vi "Gas-Control-GUI-v2.vi"() -> ()   [LabVIEW 2021]
uses:
  Controls/AR-Auto-Fill.ctl
  Controls/AR-Auto-Purge.ctl
  Controls/AR-DO-Action.ctl
panel:
  in  "Tab Control":enum32{"INDICATORS", "CHART"}(tab)
  out "Vac sol timer":dbl caption="Vac Solenoid Timer" format="%.1f sec"
  out "Gas sol timer":dbl caption="Gas Solenoid Timer" format="%.1f sec"
  out "O2 Timer":dbl format="%.1f sec"
  out "10 Torr (AI0)":dbl=10.152873763511888 caption="10 Torr Gage" format="%.3f Torr"
  out "1000 Torr (AI1)":dbl=821.8018332044094 caption="1000 Torr Gage" format="%.2f Torr"
  out "O2 1000ppm (AI3)":dbl=-245.94695681089067 caption="1000 PPM O2" format="%.0f PPM"
  out "0-25% O2 (AI2)":dbl=-6.135249063386897 caption="0-25% O2" format="%.2f %"
  in  "Full Ar Limit Torr":dbl=850.0 format="%#_13g"
  in  "Pump Down Limit Torr":dbl=320.0 format="%#_13g"
  in  "Partial Ar Fill Limit Torr":dbl=750.0 format="%#_13g"
  in  "Number of cycles":i32=25
  out "Cycle Timer":dbl format="%.1f sec"
  out "Completed Cycles":i32
  out "Pressure/O2":T1(graph) caption="Waveform Chart - Light"
  out "error out":errorcluster
  out "Log Written":bool=TRUE
  in  "Every X sec":dbl=60.0
  in  "Path to Save Report":path=path "C:/Users/cleanroom/Desktop/Gas-cycle-logs/Cycles-11-9-(750T-24cyc).csv"
  in  "LOG":bool
  out "Data":bool[](array[boolean])=[FALSE, FALSE, TRUE]
  in  "1000T Sim 2":dbl=1.0
  in  ">750 sim 2":bool=TRUE
  in  "10T Sim 2":dbl=10.0
  in  "<0.1T sim 2":bool
  out "Purge State":T2
  in  "simulate":bool
  out "Fill State":T3
  out "O2 pwr":bool
  out "Gas SOL":bool
  out "Vac SOL":bool
  in  "Quit":bool
  out "Purge Done":bool
  in  "Auto purge":bool
  out "Gage Err (DI2)":bool
  in  "O2 1000ppm (DO3)":bool
  in  "Gas sol (DO2)":bool
  in  "Vac sol (DO1)":bool
  in  "Pump (DO0)":bool
  out "Fill Done":bool
  in  "Auto fill":bool
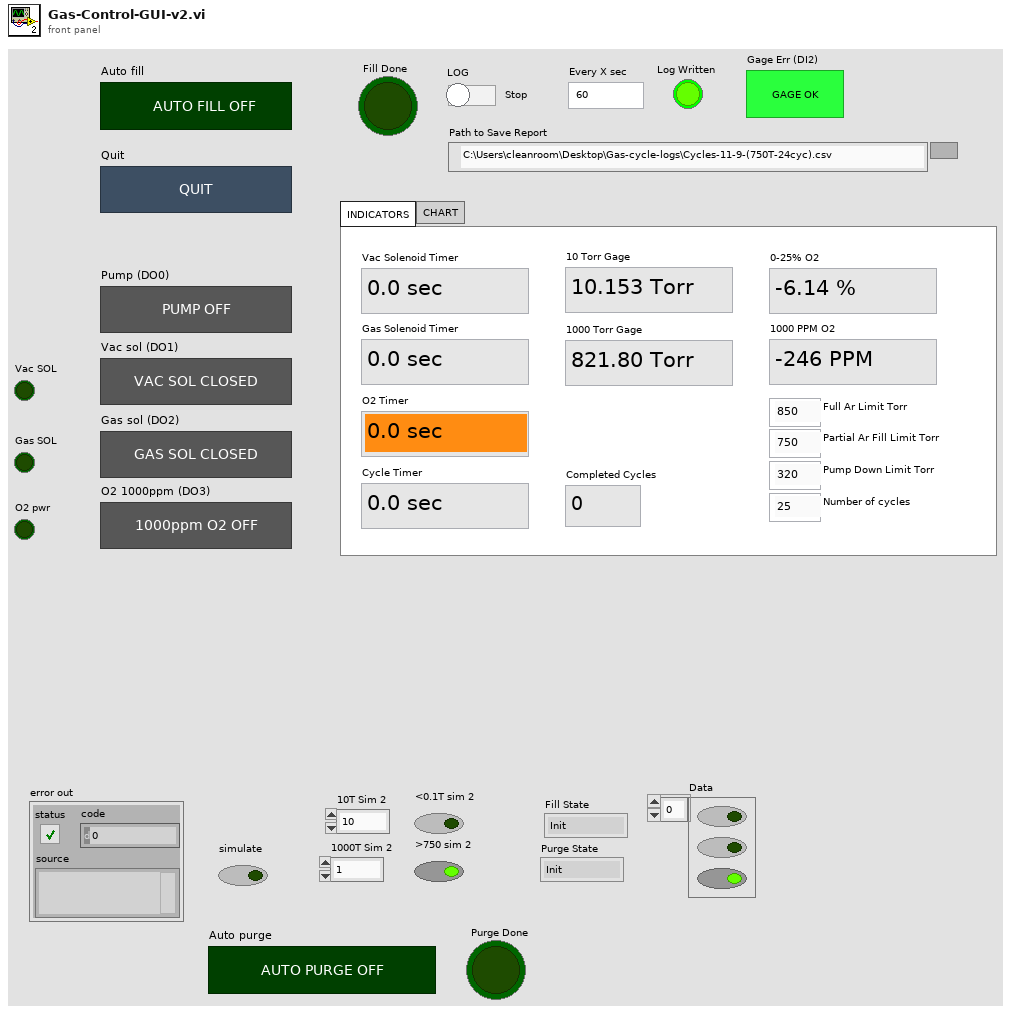
[diagram p1: front panel]
types:
  T1 = cluster{"1000 Torr (AI1)":dbl, "O2 1000ppm (AI3)":dbl}
  T2 = typedef "AR-Auto-Purge.ctl" = enum16{"Init", "Start Pump", "Stop Pump", "10T Gage", "1000T Gage", "End"}
  T3 = typedef "AR-Auto-Fill.ctl" = enum16{"Init", "Start Pump", "Stop Pump", "Gas Open", "Gas Close", "10T Gage", "1000T Gage", "End", "Vac Open", "Vac Close", "Decide"}
  T4 = typedef "AR-DO-Action.ctl" = enum16{"Init", "Update", "Keep DO3"}
  T5 = enum8{"Enabled", "Disabled", "Disabled and Grayed Out"}
  T6 = cluster{"10 Torr (AI0)":dbl, "1000 Torr (AI1)":dbl, "0-25% O2 (AI2)":dbl, "O2 1000ppm (AI3)":dbl, "Vac sol timer":dbl, "Gas sol timer":dbl, "O2 Timer":dbl, "Vac SOL":bool, "Gas SOL":bool, "O2 1000ppm (DO3)":bool}
  T7 = cluster{"1000 Torr (AI1)":dbl, "O2 1000ppm (AI3)":dbl}[]
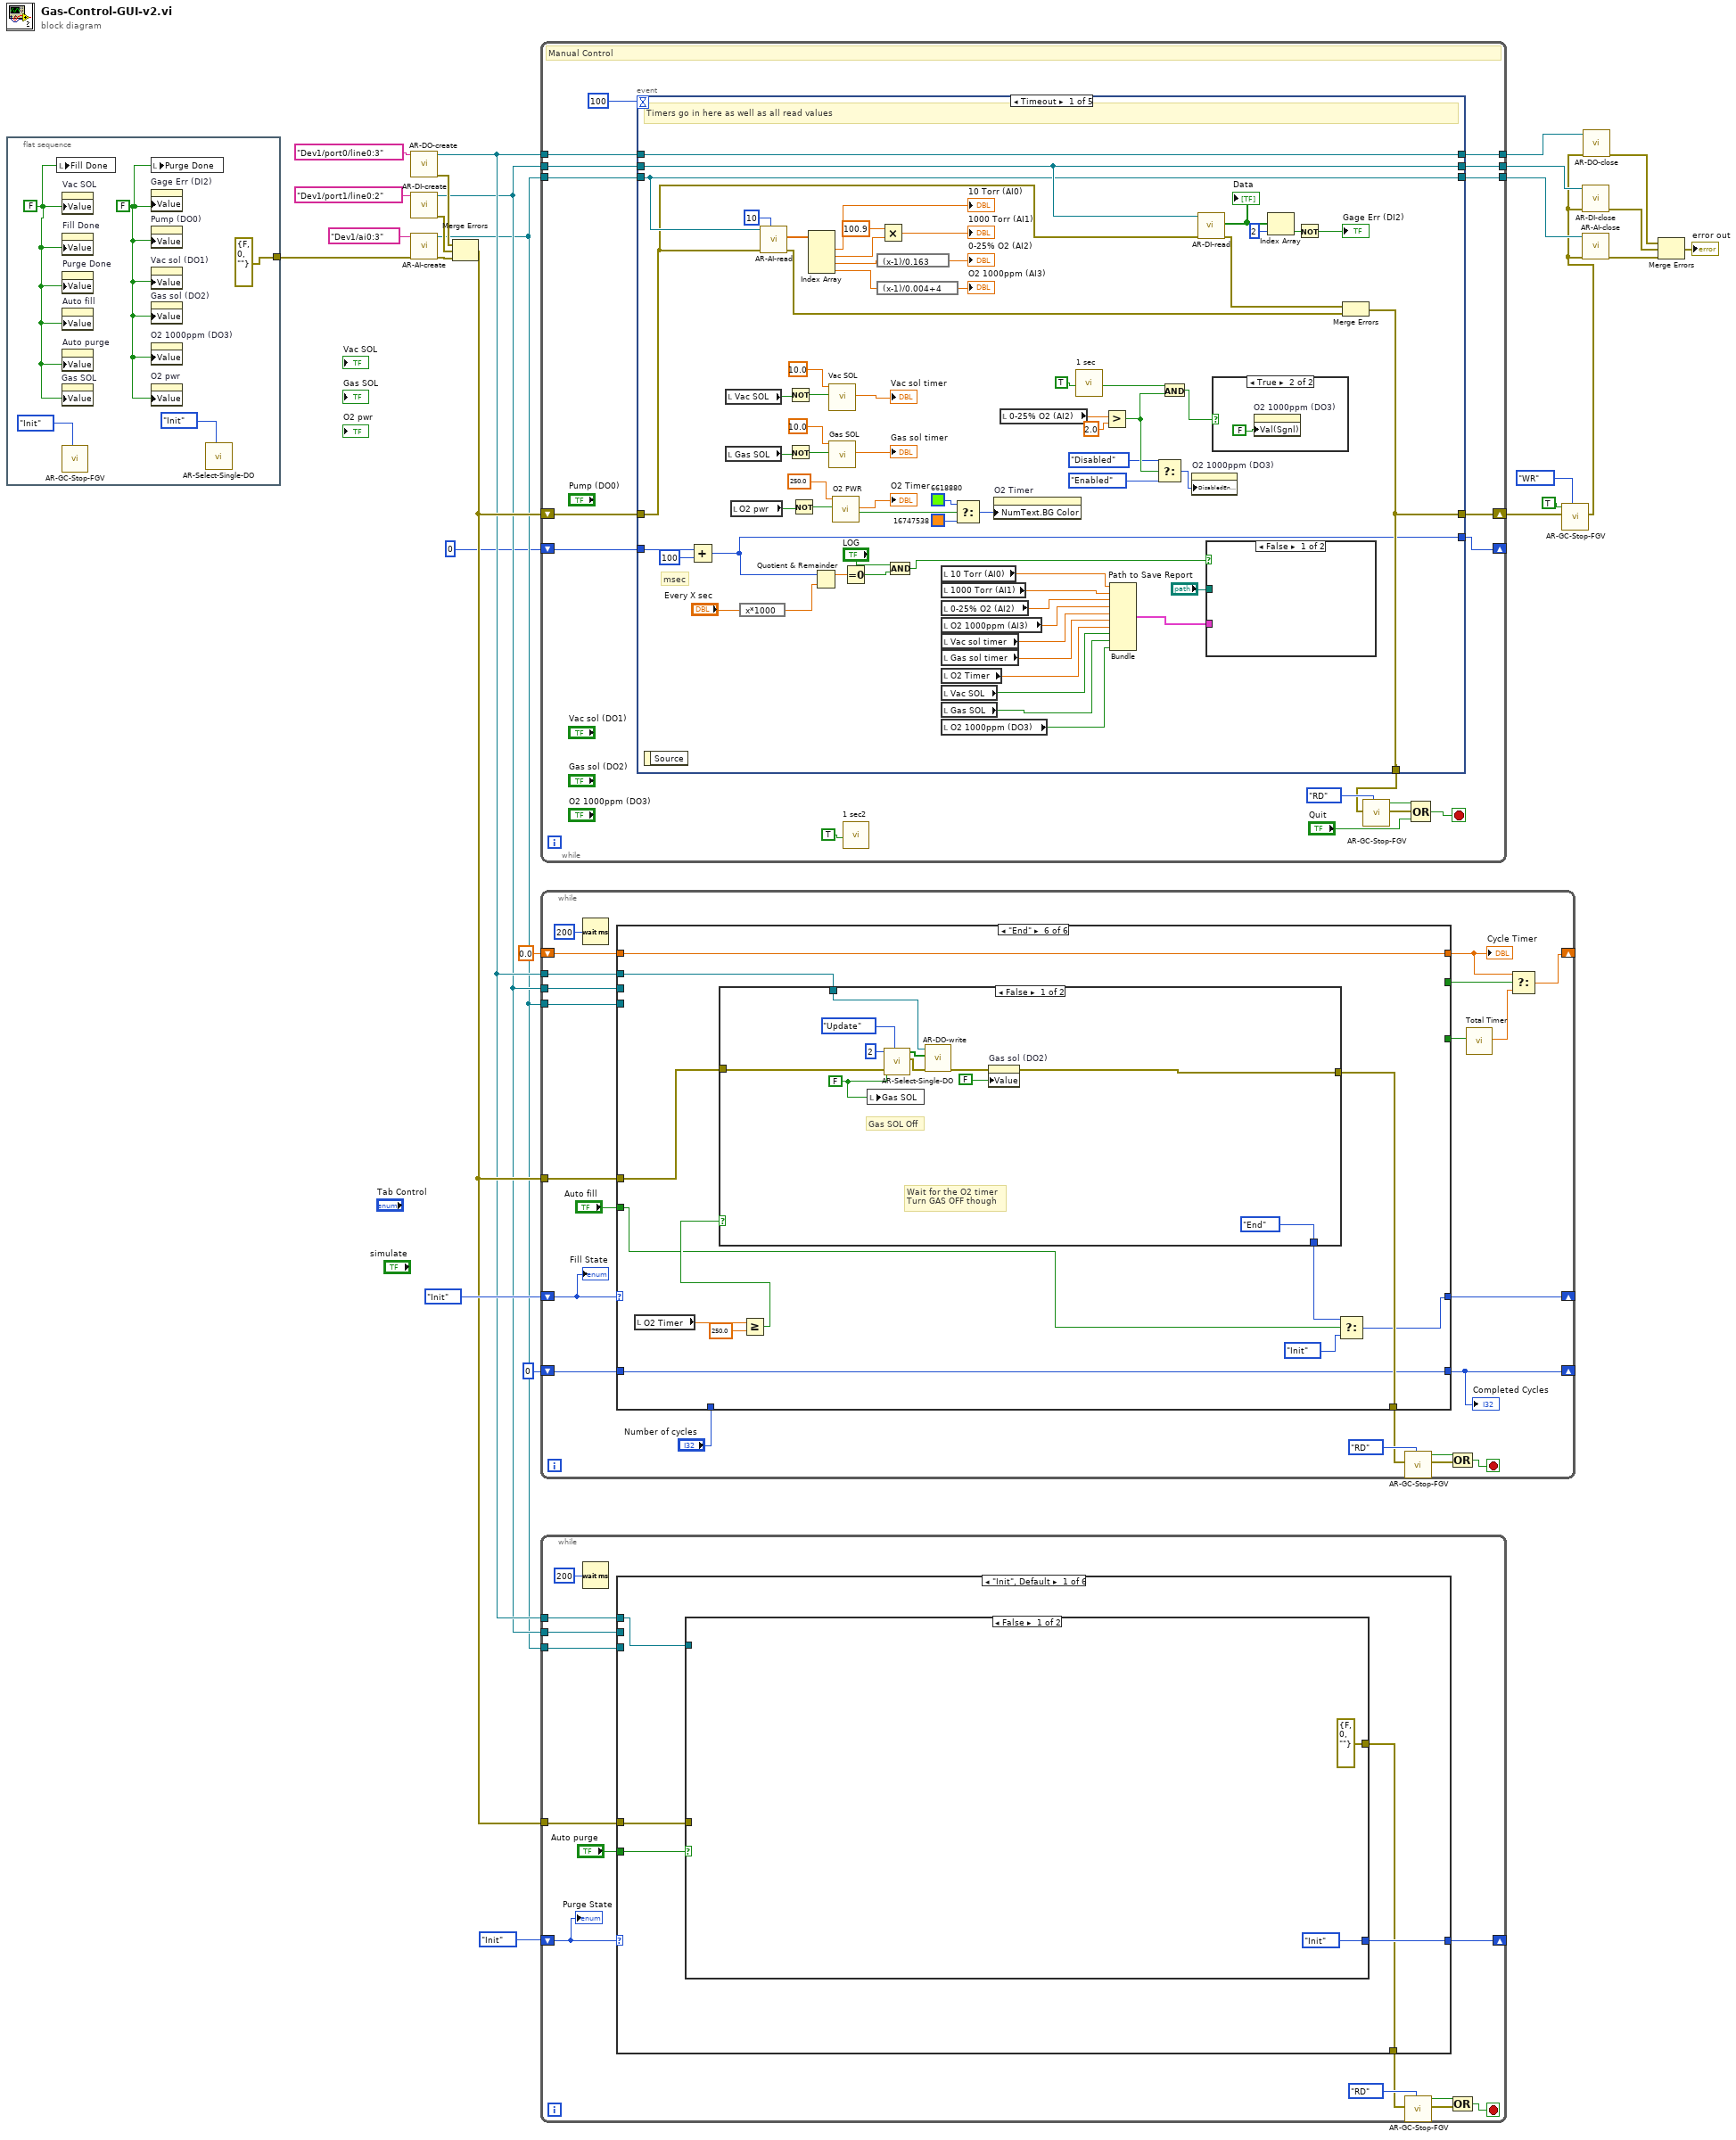
[diagram p0: block diagram]
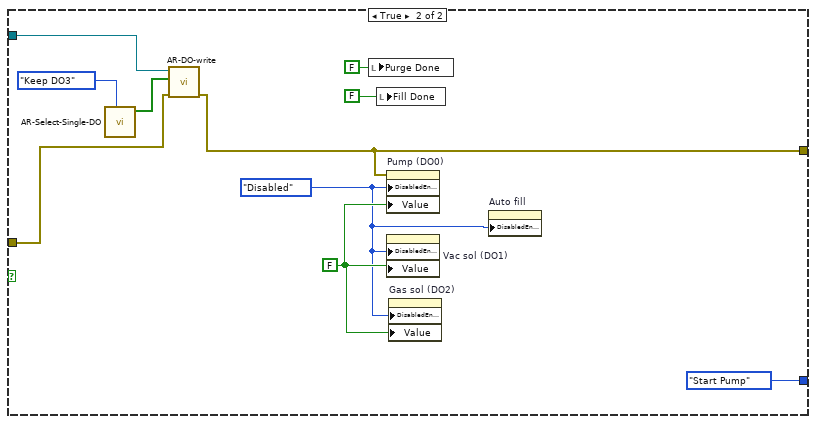
[diagram p2: hidden frame]
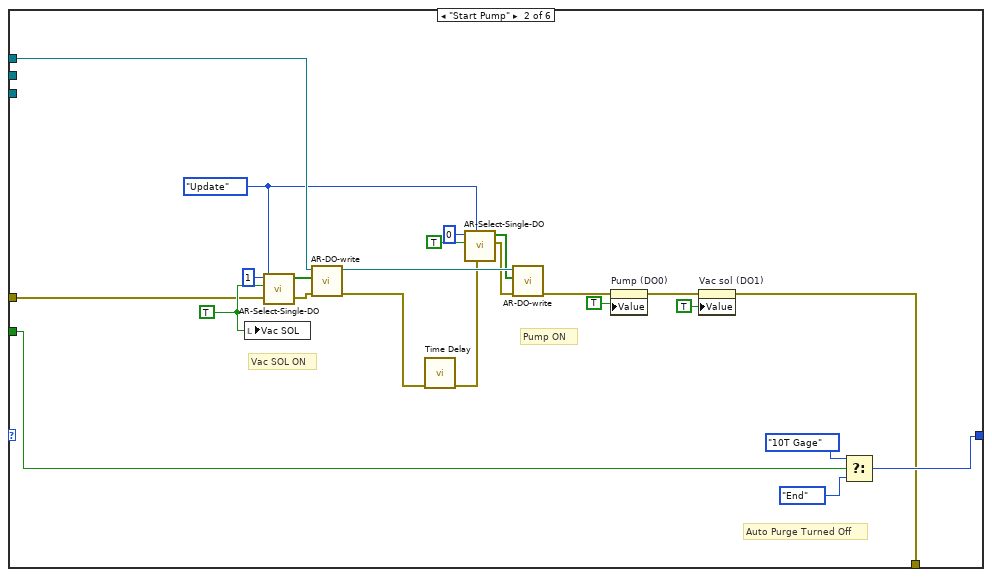
[diagram p3: hidden frame]
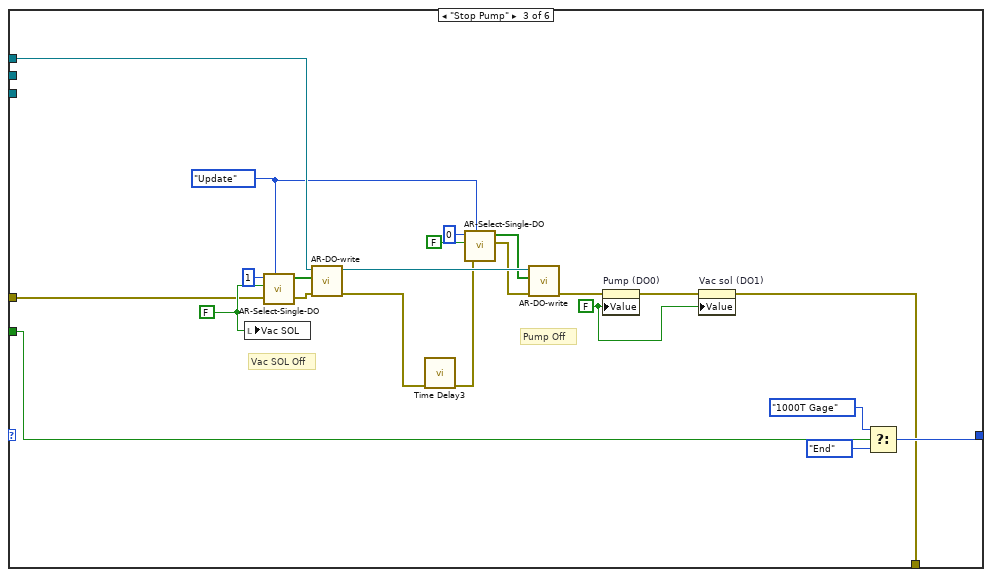
[diagram p4: hidden frame]
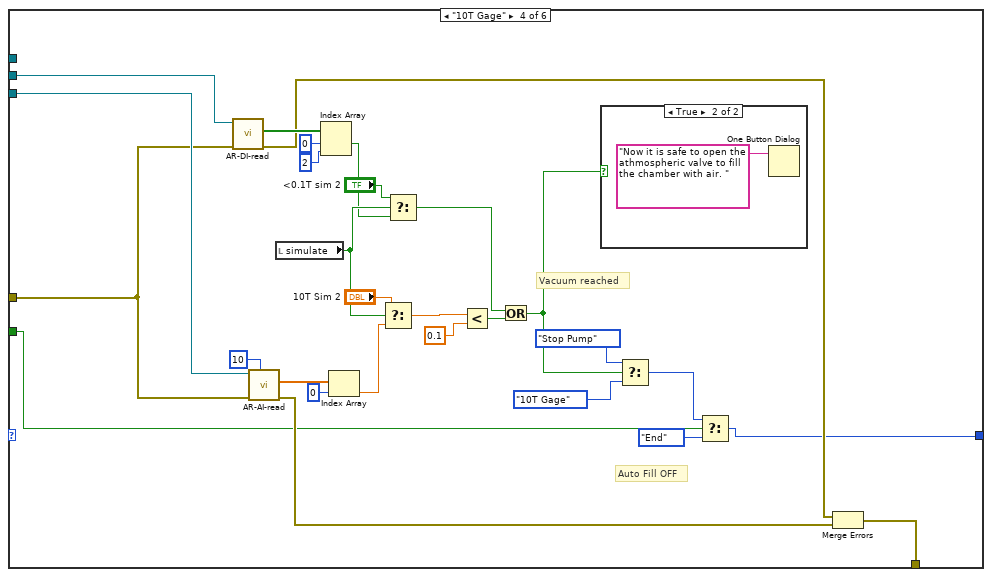
[diagram p5: hidden frame]
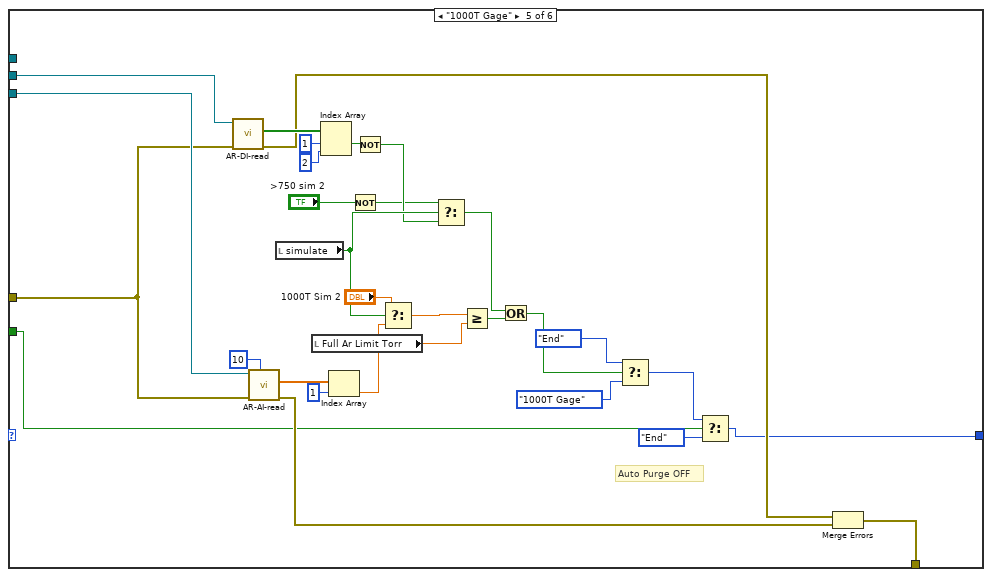
[diagram p7: hidden frame]
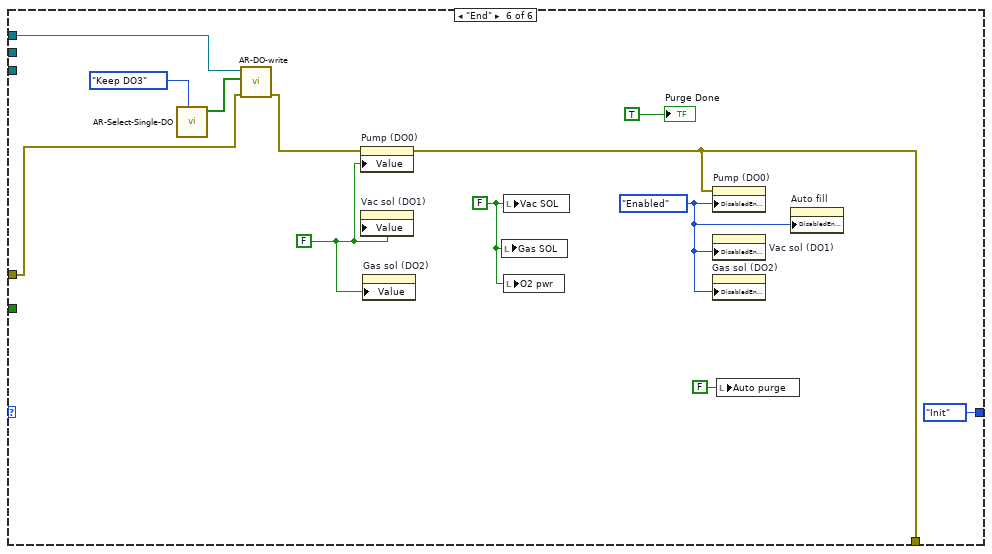
[diagram p8: hidden frame]
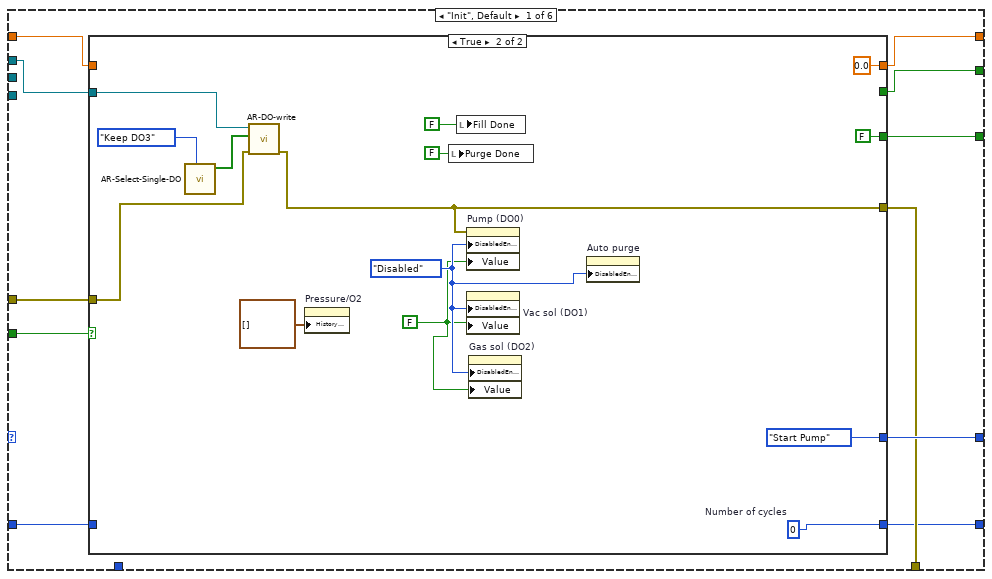
[diagram p9: hidden frame]
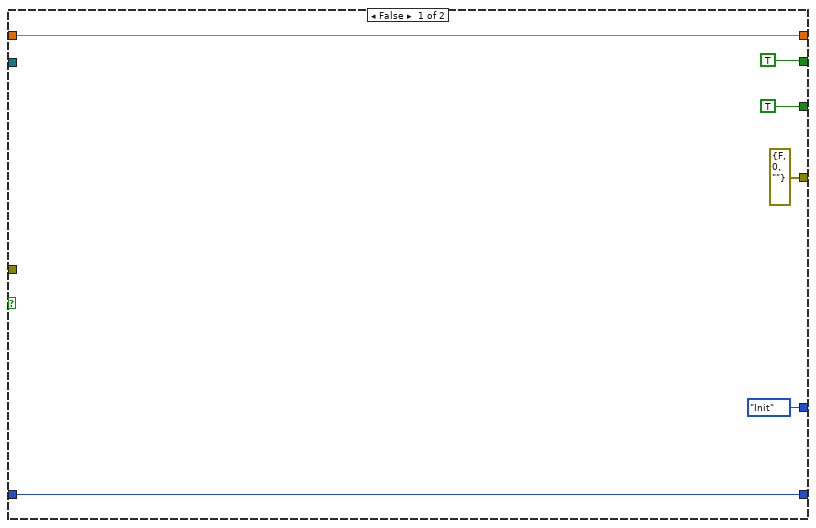
[diagram p10: hidden frame]
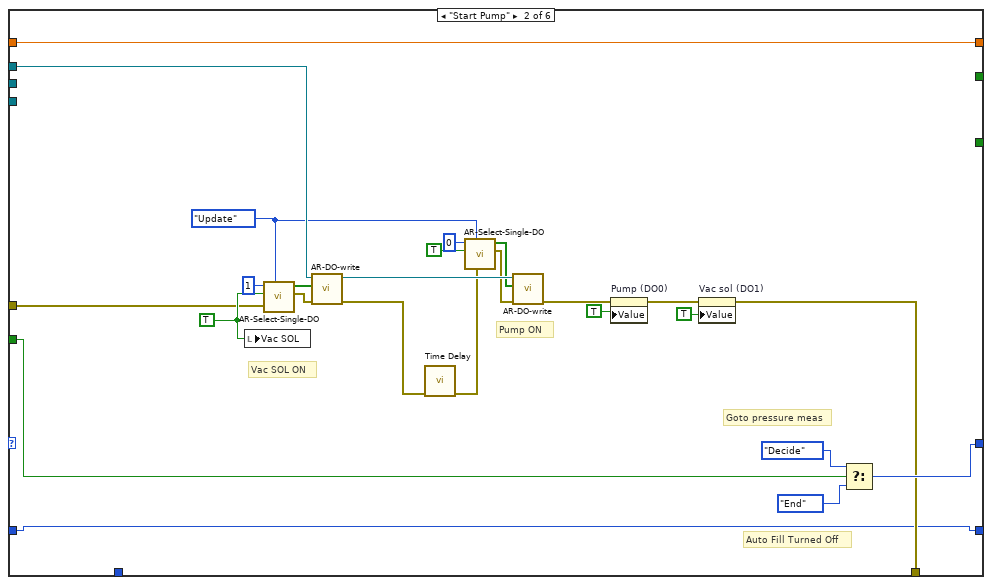
[diagram p11: hidden frame]
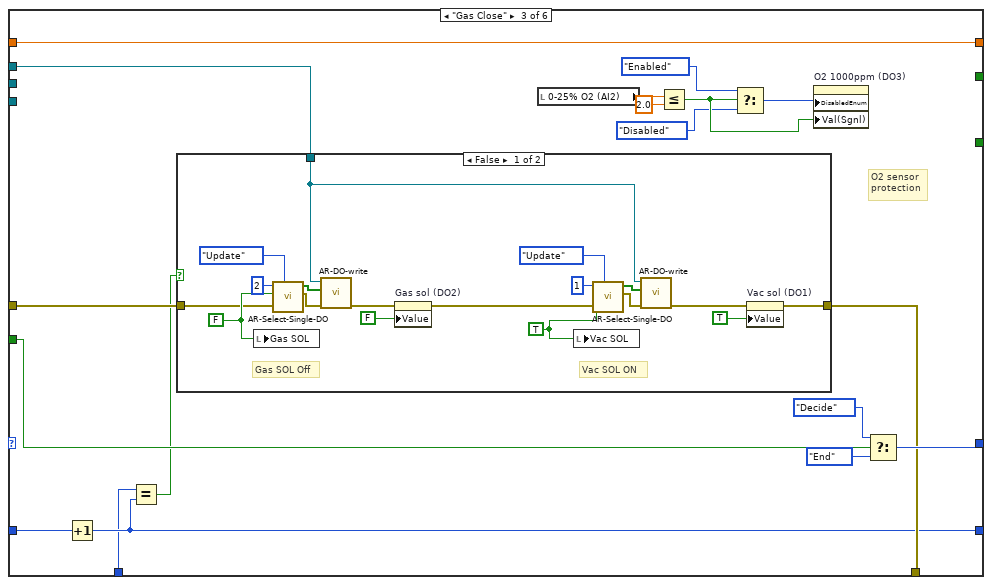
[diagram p12: hidden frame]
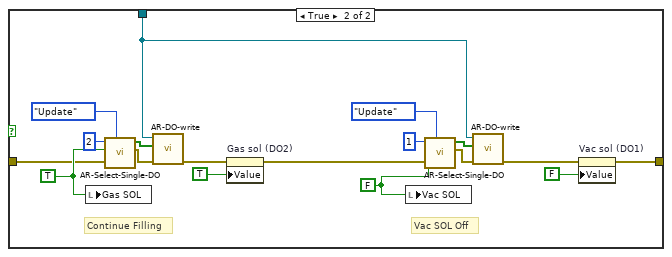
[diagram p13: hidden frame]
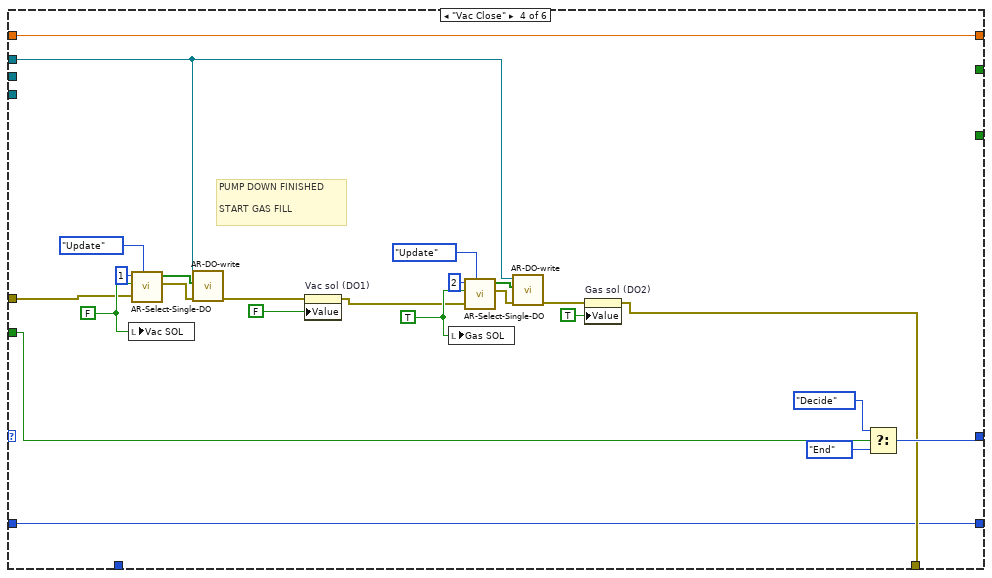
[diagram p14: hidden frame]
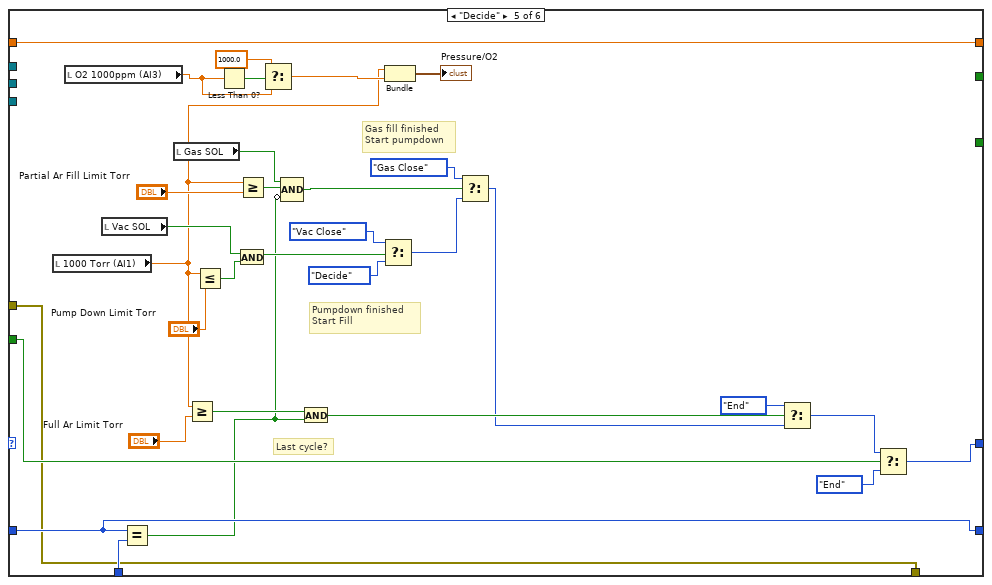
[diagram p15: hidden frame]
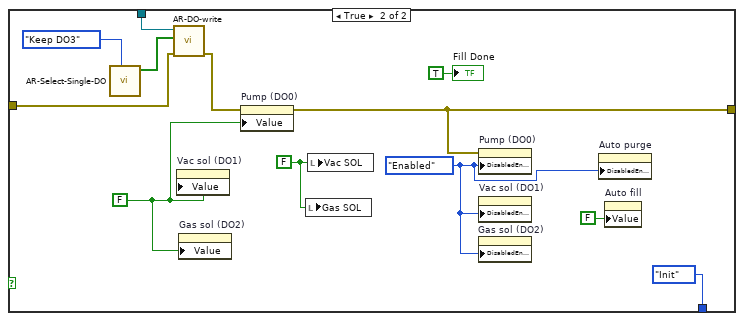
[diagram p16: hidden frame]
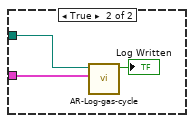
[diagram p18: hidden frame]
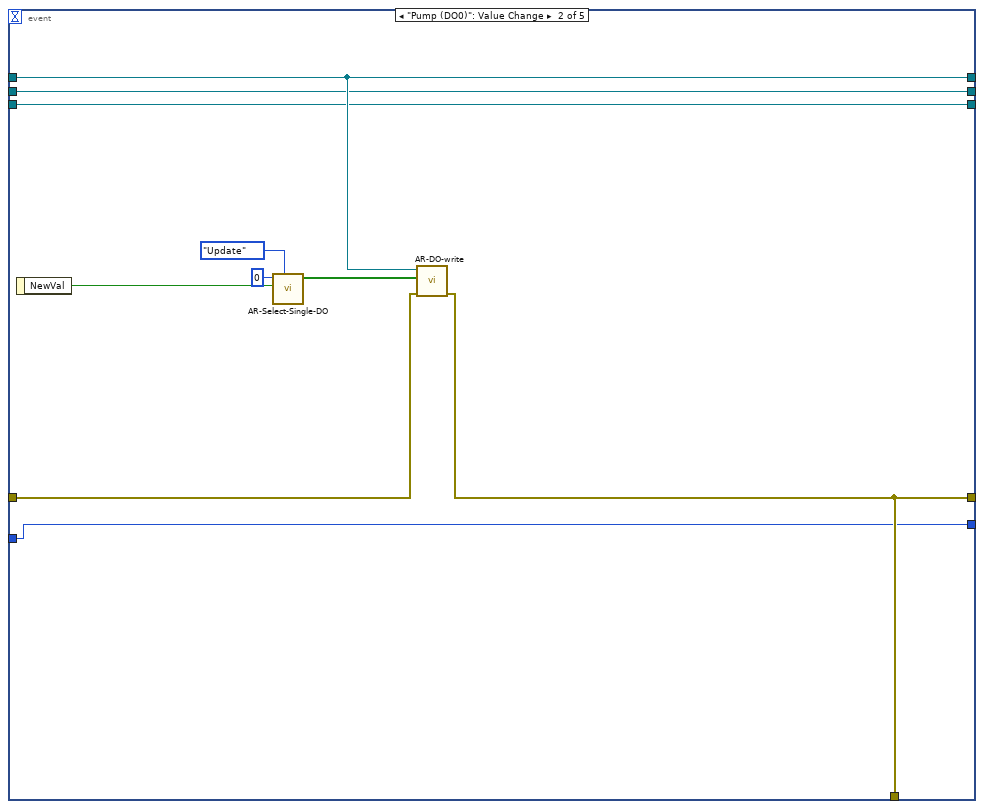
[diagram p19: hidden frame]
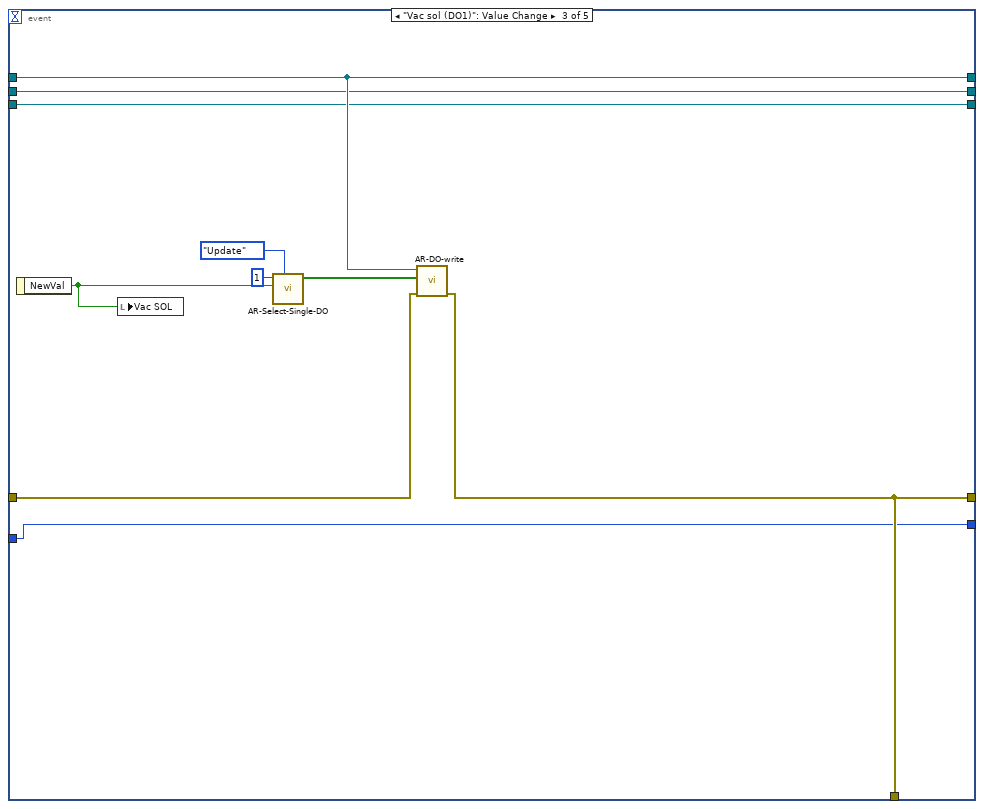
[diagram p20: hidden frame]
diagram:
  n1 = flat-sequence {
    tunnel: [errorcluster {"status"=FALSE, "code"=0, "source"=""} ("error out")] -> w15
    frame #0 {
      w29 = FALSE ("Vac SOL")
      w30 = FALSE ("Vac SOL")
      n2 = local write "Fill Done"(w30) -> ()
      n3 = property on="Vac SOL" class="Bool (strict)"("Value"=w30) -> ()  [unwired: 2 in, 2 out]
      n4 = property on="Fill Done" class="Bool (strict)"("Value"=w30) -> ()  [unwired: 2 in, 2 out]
      n5 = property on="Purge Done" class="Bool (strict)"("Value"=w30) -> ()  [unwired: 2 in, 2 out]
      n6 = property on="Auto fill" class="Bool (strict)"("Value"=w30) -> ()  [unwired: 2 in, 2 out]
      n7 = property on="Auto purge" class="Bool (strict)"("Value"=w30) -> ()  [unwired: 2 in, 2 out]
      n8 = property on="Gas SOL" class="Bool (strict)"("Value"=w30) -> ()  [unwired: 2 in, 2 out]
      n9 = call "AR-GC-Stop-FGV.vi"("Action (RD)"=enum16{"Init", "WR", "RD"}."Init") -> ()  [unwired: 9 in, 2 out]
      n10 = local write "Purge Done"(w29) -> ()
      n11 = property on="Gage Err (DI2)" class="Bool"("Value"=w29) -> ()  [unwired: 2 in, 2 out]
      n12 = property on="Pump (DO0)" class="Bool (strict)"("Value"=w29) -> ()  [unwired: 2 in, 2 out]
      n13 = property on="Vac sol (DO1)" class="Bool (strict)"("Value"=w29) -> ()  [unwired: 2 in, 2 out]
      n14 = property on="Gas sol (DO2)" class="Bool (strict)"("Value"=w29) -> ()  [unwired: 2 in, 2 out]
      n15 = property on="O2 1000ppm (DO3)" class="Bool (strict)"("Value"=w29) -> ()  [unwired: 2 in, 2 out]
      n16 = property on="O2 pwr" class="Bool (strict)"("Value"=w29) -> ()  [unwired: 2 in, 2 out]
      n17 = call "AR-Select-Single-DO.vi"("Action"=AR-DO-Action."Init") -> ()  [unwired: 9 in, 2 out]
    }
  }
  n18 = call "AR-DO-create.vi"("lines"=tag "Dev1/port0/line0:3") -> ("error out"=w18:errorcluster, "DO task out"=w8:refnum<k21>)  [unwired: 9 in]
  n19 = call "AR-DI-create.vi"("lines"=tag "Dev1/port1/line0:2") -> ("error out"=w17:errorcluster, "DI task out"=w7:refnum<k21>)  [unwired: 9 in]
  n20 = call "AR-AI-create.vi"("error in"=w15, "lines"=tag "Dev1/ai0:3") -> ("error out"=w16:errorcluster, "AI task out"=w6:refnum<k21>)  [unwired: 8 in]
  n21 = Merge Errors(w18, w17, w16) -> (w9:errorcluster)
  n22 = while {
    tunnel: w8 -> [w50]
    tunnel: w7 -> [w49]
    tunnel: w6 -> [w48]
    shift-right: [w47] -> w12
    shift-left: w9 -> [w46]
    tunnel: [w43] -> w24
    tunnel: [w42] -> w23
    tunnel: [w41] -> w22
    shift-right: [w35] -> _
    shift-left: 0 -> [w34]
    stop <- w45 stop-if-true
    # "Manual Control"
    n23 = event shown="[0] Timeout" {
      selector: _ -> [_ _ _ _ _]
      dyn-events: _ -> [_ _ _ _ _]
      timeout: 100 -> [_ _ _ _ _]
      tunnel: w50 -> [w108 w125 w136 w146 w156]
      tunnel: w49 -> [w107 w124 w135 w145 w155]
      tunnel: w48 -> [w106 w123 w134 w144 w154]
      tunnel: [w105 w126 w137 w147 w157] -> w47
      tunnel: w46 -> [w103 w127 w138 w148 w158]
      tunnel: [w105 w126 w137 w147 w157] -> w39
      tunnel: [w108 w125 w136 w146 w156] -> w43
      tunnel: [w107 w124 w135 w145 w155] -> w42
      tunnel: [w106 w123 w134 w144 w154] -> w41
      tunnel: w34 -> [w80 w122 w132 w142 w152]
      tunnel: [w66 w122 w132 w142 w152] -> w35
      event Timeout {
        # "msec"
        # "Timers go in here as well as all read values"
        n24 = event-data() -> ()  [unwired: 1 in, 1 out]
        n25 = Add(x=w80, y=100) -> (x+y=w66:i32)
        n26 = local read "Vac SOL"() -> (w116:bool)
        n27 = local read "Gas SOL"() -> (w101:bool)
        n28 = local read "O2 pwr"() -> (w97:bool)
        n29 = expression code="x*1000"("Every X sec") -> (w76:dbl)
        n30 = call "AR-AI-read.vi"("number of samples"=10, "error in"=w103, "AI task in"=w106) -> ("error out"=w83:errorcluster, "Data"=w111:dbl[])  [unwired: 6 in, 1 out]
        n31 = Not(x=w116) -> (.not. x?=w117:bool)
        n32 = Not(x=w101) -> (.not. x?=w100:bool)
        n33 = Not(x=w97) -> (.not. x?=w98:bool)
        n34 = Index Array(array=w111) -> (element #1=→"10 Torr (AI0)":dbl, element #2=w90:dbl, element #3=w87:dbl, element #4=w84:dbl)  [unwired: 4 in]
        n35 = Quotient & Remainder(x=w66, y=w76) -> (x-y*floor(x/y)=w77:dbl)  [unwired: 1 out]
        n36 = call "Vac SOL"("Time Target (s)"=10.0, "Reset"=w117) -> ("Elapsed Time (s)"=→"Vac sol timer":dbl)  [unwired: 10 in, 7 out]
        n37 = call "Gas SOL"("Time Target (s)"=10.0, "Reset"=w100) -> ("Elapsed Time (s)"=→"Gas sol timer":dbl)  [unwired: 10 in, 7 out]
        n38 = call "O2 PWR"("Time Target (s)"=250.0, "Reset"=w98) -> ("Elapsed Time (s)"=→"O2 Timer":dbl, "Time has Elapsed"=w93:bool)  [unwired: 10 in, 6 out]
        n39 = Equal To 0?(x=w77) -> (x = 0?=w74:bool)
        n40 = expression code="(x-1)/0.163"(w87) -> (→"0-25% O2 (AI2)":dbl)
        n41 = expression code="(x-1)/0.004+4"(w84) -> (→"O2 1000ppm (AI3)":dbl)
        n42 = Multiply(x=100.9, y=w90) -> (x*y=→"1000 Torr (AI1)":dbl)
        n43 = And(x="LOG", y=w74) -> (x .and. y?=w67:bool)
        n44 = local read "10 Torr (AI0)"() -> (w72:dbl)
        n45 = local read "1000 Torr (AI1)"() -> (w71:dbl)
        n46 = local read "0-25% O2 (AI2)"() -> (w70:dbl)
        n47 = local read "O2 1000ppm (AI3)"() -> (w69:dbl)
        n48 = local read "Vac sol timer"() -> (w65:dbl)
        n49 = local read "Gas sol timer"() -> (w64:dbl)
        n50 = local read "O2 Timer"() -> (w63:dbl)
        n51 = local read "Vac SOL"() -> (w62:bool)
        n52 = local read "Gas SOL"() -> (w61:bool)
        n53 = local read "O2 1000ppm (DO3)"() -> (w60:bool)
        n54 = Select(t=u32 6618880 ("Numeric Text.Colors:BG Color"), s=w93, f=u32 16747538 ("Numeric Text.Colors:BG Color")) -> (s? t:f=w91:u32)
        n55 = property on="O2 Timer" class="DigNum (strict)"("NumText.BG Color"=w91) -> ()  [unwired: 2 in, 2 out]
        n56 = local read "0-25% O2 (AI2)"() -> (w58:dbl)
        n57 = call "1 sec"("Auto Reset"=TRUE) -> ("Time has Elapsed"=w56:bool)  [unwired: 11 in, 7 out]
        n58 = Greater?(x=w58, y=2.0) -> (0:w54:bool)
        n59 = Bundle("10 Torr (AI0)"=w72, "1000 Torr (AI1)"=w71, "0-25% O2 (AI2)"=w70, "O2 1000ppm (AI3)"=w69, "Vac sol timer"=w65, "Gas sol timer"=w64, "O2 Timer"=w63, "Vac SOL"=w62, "Gas SOL"=w61, "O2 1000ppm (DO3)"=w60) -> (w68:T6)  [unwired: 1 in]
        n60 = Select(t=T5."Disabled" ("Disabled"), s=w54, f=T5."Enabled" ("Disabled")) -> (s? t:f=w51:T5)
        n61 = And(x=w56, y=w54) -> (x .and. y?=w55:bool)
        n62 = property on="O2 1000ppm (DO3)" class="Bool (strict)"("DisabledEnum"=w51) -> ()  [unwired: 2 in, 2 out]
        n63 = call "AR-DI-read.vi"("error in"=w103, "DI task in"=w107) -> ("error out"=w109:errorcluster, "Data"=w114:bool[])  [unwired: 7 in, 1 out]
        "Data" <- w114
        n64 = case shown="False" w67 {
          tunnel: "Path to Save Report" -> [_ w121]
          tunnel: w68 -> [_ w119]
          frame False {
          }
          frame True {
            n65 = call "AR-Log-gas-cycle.vi"("Log Data"=w119, "Path to Save Report"=w121) -> ("Log Written"=→"Log Written":bool)  [unwired: 8 in, 1 out]
          }
        }
        n66 = case shown="True" w55 {
          frame False {
          }
          frame True {
            n67 = property on="O2 1000ppm (DO3)" class="Bool (strict)"("Val(Sgnl)"=FALSE ("Value (Signaling)")) -> ()  [unwired: 2 in, 2 out]
          }
        }
        n68 = Index Array(array=w114, index=2) -> (element=w82:bool)
        n69 = Not(x=w82) -> (.not. x?=→"Gage Err (DI2)":bool)
        n70 = Merge Errors(w109, w83) -> (w105:errorcluster)
      }
      event "Pump (DO0)": Value Change {
        n71 = event-data() -> ("NewVal"=w128:bool)  [unwired: 1 in]
        n72 = call "AR-Select-Single-DO.vi"("Action"=enum16{"Init", "Update"}."Update", "DO"=w128, "index"=0) -> ("DO Data"=w130:bool[])  [unwired: 7 in, 1 out]
        n73 = call "AR-DO-write.vi"("error in (no error)"=w127, "Data"=w130, "DO task in"=w125) -> ("error out"=w126:errorcluster)  [unwired: 7 in, 1 out]
      }
      event "Vac sol (DO1)": Value Change {
        n74 = event-data() -> ("NewVal"=w133:bool)  [unwired: 1 in]
        n75 = local write "Vac SOL"(w133) -> ()
        n76 = call "AR-Select-Single-DO.vi"("Action"=enum16{"Init", "Update"}."Update", "DO"=w133, "index"=1) -> ("DO Data"=w140:bool[])  [unwired: 7 in, 1 out]
        n77 = call "AR-DO-write.vi"("error in (no error)"=w138, "Data"=w140, "DO task in"=w136) -> ("error out"=w137:errorcluster)  [unwired: 7 in, 1 out]
      }
      event "Gas sol (DO2)": Value Change {
        n78 = event-data() -> ("NewVal"=w143:bool)  [unwired: 1 in]
        n79 = local write "Gas SOL"(w143) -> ()
        n80 = call "AR-Select-Single-DO.vi"("Action"=enum16{"Init", "Update"}."Update", "DO"=w143, "index"=2) -> ("DO Data"=w150:bool[])  [unwired: 7 in, 1 out]
        n81 = call "AR-DO-write.vi"("error in (no error)"=w148, "Data"=w150, "DO task in"=w146) -> ("error out"=w147:errorcluster)  [unwired: 7 in, 1 out]
      }
      event "O2 1000ppm (DO3)": Value Change {
        n82 = event-data() -> ("NewVal"=w153:bool)  [unwired: 1 in]
        n83 = local write "O2 pwr"(w153) -> ()
        n84 = call "AR-Select-Single-DO.vi"("Action"=enum16{"Init", "Update"}."Update", "DO"=w153, "index"=3) -> ("DO Data"=w160:bool[])  [unwired: 7 in, 1 out]
        n85 = call "AR-DO-write.vi"("error in (no error)"=w158, "Data"=w160, "DO task in"=w156) -> ("error out"=w157:errorcluster)  [unwired: 7 in, 1 out]
      }
    }
    n86 = call "1 sec2"("Auto Reset"=TRUE) -> ()  [unwired: 11 in, 8 out]
    n87 = call "AR-GC-Stop-FGV.vi"("Action (RD)"=enum16{"Init", "WR", "RD"}."RD", "error in"=w39) -> ("error out"=w38:errorcluster, "Out"=w37:bool)  [unwired: 8 in]
    n88 = Compound Arithmetic op=OR(w37, w38, "Quit") -> (w45:bool)
  }
  n89 = while {
    tunnel: w8 -> [w175]
    tunnel: w7 -> [w171]
    tunnel: w6 -> [w172]
    shift-right: [w177] -> _
    shift-left: AR-Auto-Fill."Init" ("Fill State") -> [w176]
    tunnel: w9 -> [w173]
    shift-right: [w162] -> _
    shift-left: 0 ("Number of cycles") -> [w170]
    shift-right: [w163] -> _
    shift-left: 0.0 ("Elapsed Time (s)") -> [w167]
    stop <- w180 stop-if-true
    n90 = Wait (ms)(milliseconds to wait=u32 200) -> ()  [unwired: 1 out]
    n91 = case shown="\"End\"" w176 {
      tunnel: "Auto fill" -> [w194 w230 w257 w314 w332 w353]
      tunnel: [w193 w227 w254 w311 w329 w350] -> w177
      tunnel: w175 -> [w192 w237 w248 w295 _ w361]
      tunnel: [w191 w222 w252 w301 w327 w359] -> w174
      tunnel: w173 -> [w190 w217 w249 w299 w327 w360]
      tunnel: w172 -> [_ _ _ _ _ _]
      tunnel: w171 -> [_ _ _ _ _ _]
      tunnel: [w189 w218 w251 w300 w328 w358] -> w162
      tunnel: w170 -> [w188 w218 w253 w300 w328 w358]
      tunnel: "Number of cycles" -> [_ _ w250 _ w337 _]
      tunnel: [w187 _ _ _ _ _] -> w168
      tunnel: w167 -> [w186 w215 w246 w294 w325 w357]
      tunnel: [w185 w215 w246 w294 w325 w357] -> w165
      tunnel: [w184 _ _ _ _ _] -> w166
      frame "Init", Default {
        n92 = case shown="True" w194 {
          tunnel: [AR-Auto-Fill."Init" ("Fill State") AR-Auto-Fill."Start Pump" ("Fill State")] -> w193
          tunnel: w192 -> [_ w212]
          tunnel: [errorcluster {"status"=FALSE, "code"=0, "source"=""} ("error out") w208] -> w191
          tunnel: w190 -> [_ w210]
          tunnel: [w198 w204] -> w189
          tunnel: w188 -> [w198 _]
          tunnel: [TRUE FALSE] -> w187
          tunnel: w186 -> [w196 _]
          tunnel: [w196 0.0 ("Elapsed Time (s)")] -> w185
          tunnel: [TRUE _] -> w184
          frame False {
          }
          frame True {
            w204 = 0  # Number of cycles
            w209 = FALSE
            w214 = T5."Disabled" ("Disabled")
            n93 = call "AR-Select-Single-DO.vi"("Action"=AR-DO-Action."Keep DO3") -> ("DO Data"=w211:bool[])  [unwired: 9 in, 1 out]
            n94 = call "AR-DO-write.vi"("error in (no error)"=w210, "Data"=w211, "DO task in"=w212) -> ("error out"=w208:errorcluster)  [unwired: 7 in, 1 out]
            n95 = property on="Pressure/O2" class="WFChart (strict)"("History Data"=T7 []) -> ()  [unwired: 2 in, 2 out]
            n96 = local write "Purge Done"(FALSE ("Purge Done")) -> ()
            n97 = local write "Fill Done"(FALSE ("Purge Done")) -> ()
            n98 = property on="Pump (DO0)" class="Bool (strict)"(error in=w208, "DisabledEnum"=w214, "Value"=w209) -> ()  [unwired: 1 in, 2 out]
            n99 = property on="Vac sol (DO1)" class="Bool (strict)"("DisabledEnum"=w214, "Value"=w209) -> ()  [unwired: 2 in, 2 out]
            n100 = property on="Gas sol (DO2)" class="Bool (strict)"("DisabledEnum"=w214, "Value"=w209) -> ()  [unwired: 2 in, 2 out]
            n101 = property on="Auto purge" class="Bool (strict)"("DisabledEnum"=w214) -> ()  [unwired: 2 in, 2 out]
          }
        }
      }
      frame "Start Pump" {
        w219 = AR-DO-Action."Update" ("Action")
        w236 = TRUE ("DO")
        # "Goto pressure meas"
        # "Auto Fill Turned Off"
        # "Pump ON"
        # "Vac SOL ON"
        n102 = local write "Vac SOL"(w236) -> ()
        n103 = call "AR-Select-Single-DO.vi"("error in (no error)"=w217, "Action"=w219, "DO"=w236, "index"=1) -> ("error out"=w216:errorcluster, "DO Data"=w238:bool[])  [unwired: 6 in]
        n104 = call "AR-DO-write.vi"("error in (no error)"=w216, "Data"=w238, "DO task in"=w237) -> ("error out"=w231:errorcluster, "DO task out"=w234:refnum<k21>)  [unwired: 7 in]
        n105 = call "Time Delay"("error in (no error)"=w231) -> ("error out"=w221:errorcluster)  [unwired: 10 in]
        n106 = call "AR-Select-Single-DO.vi"("error in (no error)"=w221, "Action"=w219, "DO"=TRUE, "index"=0) -> ("error out"=w220:errorcluster, "DO Data"=w233:bool[])  [unwired: 6 in]
        n107 = call "AR-DO-write.vi"("error in (no error)"=w220, "Data"=w233, "DO task in"=w234) -> ("error out"=w225:errorcluster)  [unwired: 7 in, 1 out]
        n108 = property on="Pump (DO0)" class="Bool (strict)"(error in=w225, "Value"=TRUE ("Pump (DO0)")) -> (error out=w224:errorcluster)  [unwired: 1 in, 1 out]
        n109 = property on="Vac sol (DO1)" class="Bool (strict)"(error in=w224, "Value"=TRUE ("Vac sol (DO1)")) -> (error out=w222:errorcluster)  [unwired: 1 in, 1 out]
        n110 = Select(t=AR-Auto-Fill."Decide" ("Fill State"), s=w230, f=AR-Auto-Fill."End" ("Fill State")) -> (s? t:f=w227:T3)
      }
      frame "Gas Close" {
        # "O2 sensor\nprotection"
        n111 = Increment(x=w253) -> (x+1=w251:i32)
        n112 = Equal?(x=w250, y=w251) -> (x = y?=w247:bool)
        n113 = case shown="False" w247 {
          tunnel: [w268 w286] -> w252
          tunnel: w249 -> [w267 w285]
          tunnel: w248 -> [w265 w283]
          frame False {
            w261 = TRUE ("DO")
            w273 = FALSE ("DO")
            # "Vac SOL ON"
            # "Gas SOL Off"
            n114 = local write "Gas SOL"(w273) -> ()
            n115 = call "AR-Select-Single-DO.vi"("error in (no error)"=w267, "Action"=AR-DO-Action."Update", "DO"=w273, "index"=2) -> ("error out"=w266:errorcluster, "DO Data"=w274:bool[])  [unwired: 6 in]
            n116 = call "AR-DO-write.vi"("error in (no error)"=w266, "Data"=w274, "DO task in"=w265) -> ("error out"=w272:errorcluster)  [unwired: 7 in, 1 out]
            n117 = property on="Gas sol (DO2)" class="Bool (strict)"(error in=w272, "Value"=FALSE ("Gas sol (DO2)")) -> (error out=w269:errorcluster)  [unwired: 1 in, 1 out]
            n118 = local write "Vac SOL"(w261) -> ()
            n119 = call "AR-Select-Single-DO.vi"("error in (no error)"=w269, "Action"=AR-DO-Action."Update", "DO"=w261, "index"=1) -> ("error out"=w258:errorcluster, "DO Data"=w264:bool[])  [unwired: 6 in]
            n120 = call "AR-DO-write.vi"("error in (no error)"=w258, "Data"=w264, "DO task in"=w265) -> ("error out"=w263:errorcluster)  [unwired: 7 in, 1 out]
            n121 = property on="Vac sol (DO1)" class="Bool (strict)"(error in=w263, "Value"=TRUE ("Gas sol (DO2)")) -> (error out=w268:errorcluster)  [unwired: 1 in, 1 out]
          }
          frame True {
            w279 = FALSE ("DO")
            w291 = TRUE ("DO")
            # "Vac SOL Off"
            # "Continue Filling"
            n122 = local write "Gas SOL"(w291) -> ()
            n123 = call "AR-Select-Single-DO.vi"("error in (no error)"=w285, "Action"=AR-DO-Action."Update", "DO"=w291, "index"=2) -> ("error out"=w284:errorcluster, "DO Data"=w292:bool[])  [unwired: 6 in]
            n124 = call "AR-DO-write.vi"("error in (no error)"=w284, "Data"=w292, "DO task in"=w283) -> ("error out"=w290:errorcluster)  [unwired: 7 in, 1 out]
            n125 = property on="Gas sol (DO2)" class="Bool (strict)"(error in=w290, "Value"=TRUE ("Gas sol (DO2)")) -> (error out=w287:errorcluster)  [unwired: 1 in, 1 out]
            n126 = local write "Vac SOL"(w279) -> ()
            n127 = call "AR-Select-Single-DO.vi"("error in (no error)"=w287, "Action"=AR-DO-Action."Update", "DO"=w279, "index"=1) -> ("error out"=w276:errorcluster, "DO Data"=w282:bool[])  [unwired: 6 in]
            n128 = call "AR-DO-write.vi"("error in (no error)"=w276, "Data"=w282, "DO task in"=w283) -> ("error out"=w281:errorcluster)  [unwired: 7 in, 1 out]
            n129 = property on="Vac sol (DO1)" class="Bool (strict)"(error in=w281, "Value"=FALSE ("Gas sol (DO2)")) -> (error out=w286:errorcluster)  [unwired: 1 in, 1 out]
          }
        }
        n130 = local read "0-25% O2 (AI2)"() -> (w244:dbl)
        n131 = Less Or Equal?(x=w244, y=2.0) -> (x <= y?=w243:bool)
        n132 = Select(t=T5."Enabled" ("Disabled"), s=w243, f=T5."Disabled" ("Disabled")) -> (s? t:f=w245:T5)
        n133 = property on="O2 1000ppm (DO3)" class="Bool (strict)"("DisabledEnum"=w245, "Val(Sgnl)"=w243) -> ()  [unwired: 2 in, 2 out]
        n134 = Select(t=AR-Auto-Fill."Decide" ("Fill State"), s=w257, f=AR-Auto-Fill."End") -> (s? t:f=w254:T3)
      }
      frame "Vac Close" {
        w306 = TRUE ("DO")
        w315 = FALSE ("DO")
        # "PUMP DOWN FINISHED\n\nSTART GAS FILL"
        n135 = local write "Vac SOL"(w315) -> ()
        n136 = call "AR-Select-Single-DO.vi"("error in (no error)"=w299, "Action"=AR-DO-Action."Update", "DO"=w315, "index"=1) -> ("error out"=w298:errorcluster, "DO Data"=w316:bool[])  [unwired: 6 in]
        n137 = call "AR-DO-write.vi"("error in (no error)"=w298, "Data"=w316, "DO task in"=w295) -> ("error out"=w309:errorcluster)  [unwired: 7 in, 1 out]
        n138 = property on="Vac sol (DO1)" class="Bool (strict)"(error in=w309, "Value"=FALSE ("Gas sol (DO2)")) -> (error out=w297:errorcluster)  [unwired: 1 in, 1 out]
        n139 = local write "Gas SOL"(w306) -> ()
        n140 = call "AR-Select-Single-DO.vi"("error in (no error)"=w297, "Action"=AR-DO-Action."Update", "DO"=w306, "index"=2) -> ("error out"=w296:errorcluster, "DO Data"=w305:bool[])  [unwired: 6 in]
        n141 = call "AR-DO-write.vi"("error in (no error)"=w296, "Data"=w305, "DO task in"=w295) -> ("error out"=w302:errorcluster)  [unwired: 7 in, 1 out]
        n142 = property on="Gas sol (DO2)" class="Bool (strict)"(error in=w302, "Value"=TRUE ("Gas sol (DO2)")) -> (error out=w301:errorcluster)  [unwired: 1 in, 1 out]
        n143 = Select(t=AR-Auto-Fill."Decide" ("Fill State"), s=w314, f=AR-Auto-Fill."End") -> (s? t:f=w311:T3)
      }
      frame "Decide" {
        # "Gas fill finished\nStart pumpdown"
        # "Last cycle?"
        # "Pumpdown finished\nStart Fill"
        n144 = local read "1000 Torr (AI1)"() -> (w320:dbl)
        n145 = local read "O2 1000ppm (AI3)"() -> (w322:dbl)
        n146 = local read "Vac SOL"() -> (w344:bool)
        n147 = Equal?(x=w328, y=w337) -> (x = y?=w326:bool)
        n148 = local read "Gas SOL"() -> (w341:bool)
        n149 = Greater Or Equal?(x=w320, y="Full Ar Limit Torr") -> (x >= y?=w335:bool)
        n150 = Less Or Equal?(x=w320, y="Pump Down Limit Torr") -> (x <= y?=w348:bool)
        n151 = Less Than 0?(x=w322) -> (x < 0?=w324:bool)
        n152 = And(x=w344, y=w348) -> (x .and. y?=w347:bool)
        n153 = Greater Or Equal?(x=w320, y="Partial Ar Fill Limit Torr") -> (x >= y?=w342:bool)
        n154 = Select(t=1000.0, s=w324, f=w322) -> (s? t:f=w321:dbl)
        n155 = Compound Arithmetic op=AND(w341, w342, invert w326) -> (w340:bool)
        n156 = And(x=w335, y=w326) -> (x .and. y?=w334:bool)
        n157 = Select(t=AR-Auto-Fill."Vac Close" ("Fill State"), s=w347, f=AR-Auto-Fill."Decide" ("Fill State")) -> (s? t:f=w338:T3)
        n158 = Bundle("1000 Torr (AI1)"=w320, "O2 1000ppm (AI3)"=w321) -> (→"Pressure/O2":T1)  [unwired: 1 in]
        n159 = Select(t=AR-Auto-Fill."Gas Close" ("Fill State"), s=w340, f=w338) -> (s? t:f=w333:T3)
        n160 = Select(t=AR-Auto-Fill."End", s=w334, f=w333) -> (s? t:f=w331:T3)
        n161 = Select(t=w331, s=w332, f=AR-Auto-Fill."End") -> (s? t:f=w329:T3)
      }
      frame "End" {
        n162 = local read "O2 Timer"() -> (w356:dbl)
        n163 = Greater Or Equal?(x=w356, y=250.0) -> (x >= y?=w354:bool)
        n164 = case shown="False" w354 {
          tunnel: w361 -> [w370 w382]
          tunnel: w360 -> [w371 w381]
          tunnel: [w369 w375] -> w359
          tunnel: [AR-Auto-Fill."End" ("Fill State") AR-Auto-Fill."Init" ("f")] -> w351
          frame False {
            w364 = FALSE ("DO")
            # "Gas SOL Off"
            # "Wait for the O2 timer\nTurn GAS OFF though"
            n165 = local write "Gas SOL"(w364) -> ()
            n166 = call "AR-Select-Single-DO.vi"("error in (no error)"=w371, "Action"=AR-DO-Action."Update", "DO"=w364, "index"=2) -> ("error out"=w366:errorcluster, "DO Data"=w368:bool[])  [unwired: 6 in]
            n167 = call "AR-DO-write.vi"("error in (no error)"=w366, "Data"=w368, "DO task in"=w370) -> ("error out"=w367:errorcluster)  [unwired: 7 in, 1 out]
            n168 = property on="Gas sol (DO2)" class="Bool (strict)"(error in=w367, "Value"=FALSE ("Gas sol (DO2)")) -> (error out=w369:errorcluster)  [unwired: 1 in, 1 out]
          }
          frame True {
            w376 = T5."Enabled" ("Disabled")
            w378 = FALSE ("Vac SOL")
            w379 = FALSE
            n169 = call "AR-Select-Single-DO.vi"("Action"=AR-DO-Action."Keep DO3") -> ("DO Data"=w383:bool[])  [unwired: 9 in, 1 out]
            n170 = call "AR-DO-write.vi"("error in (no error)"=w381, "Data"=w383, "DO task in"=w382) -> ("error out"=w380:errorcluster)  [unwired: 7 in, 1 out]
            n171 = property on="Vac sol (DO1)" class="Bool (strict)"("Value"=w379) -> ()  [unwired: 2 in, 2 out]
            n172 = property on="Gas sol (DO2)" class="Bool (strict)"("Value"=w379) -> ()  [unwired: 2 in, 2 out]
            n173 = property on="Pump (DO0)" class="Bool (strict)"(error in=w380, "Value"=w379) -> (error out=w375:errorcluster)  [unwired: 1 in, 1 out]
            n174 = local write "Gas SOL"(w378) -> ()
            n175 = local write "Vac SOL"(w378) -> ()
            n176 = property on="Pump (DO0)" class="Bool (strict)"(error in=w375, "DisabledEnum"=w376) -> ()  [unwired: 1 in, 2 out]
            n177 = property on="Vac sol (DO1)" class="Bool (strict)"("DisabledEnum"=w376) -> ()  [unwired: 2 in, 2 out]
            n178 = property on="Gas sol (DO2)" class="Bool (strict)"("DisabledEnum"=w376) -> ()  [unwired: 2 in, 2 out]
            n179 = property on="Auto purge" class="Bool (strict)"("DisabledEnum"=w376) -> ()  [unwired: 2 in, 2 out]
            n180 = property on="Auto fill" class="Bool (strict)"("Value"=FALSE ("Auto fill")) -> ()  [unwired: 2 in, 2 out]
            "Fill Done" <- TRUE ("Fill Done")
          }
        }
        n181 = Select(t=w351, s=w353, f=AR-Auto-Fill."Init" ("Fill State")) -> (s? t:f=w350:T3)
      }
    }
    "Cycle Timer" <- w165
    "Completed Cycles" <- w162
    n182 = call "AR-GC-Stop-FGV.vi"("Action (RD)"=enum16{"Init", "WR", "RD"}."RD", "error in"=w174) -> ("error out"=w182:errorcluster, "Out"=w183:bool)  [unwired: 8 in]
    n183 = Compound Arithmetic op=OR(w183, w182) -> (w180:bool)
    n184 = call "Total Timer"("Reset"=w168) -> ("Elapsed Time (s)"=w164:dbl)  [unwired: 11 in, 7 out]
    n185 = Select(t=w165, s=w166, f=w164) -> (s? t:f=w163:dbl)
    "Fill State" <- w176
  }
  n186 = while {
    tunnel: w8 -> [w390]
    tunnel: w7 -> [w386]
    tunnel: w6 -> [w387]
    shift-right: [w392] -> _
    shift-left: AR-Auto-Purge."Init" ("Purge State") -> [w391]
    tunnel: w9 -> [w388]
    stop <- w394 stop-if-true
    n187 = Wait (ms)(milliseconds to wait=u32 200) -> ()  [unwired: 1 out]
    n188 = case shown="\"Init\", Default" w391 {
      tunnel: "Auto purge" -> [w402 w426 w447 w463 w497 _]
      tunnel: [w401 w423 w444 w460 w494 AR-Auto-Purge."Init" ("f")] -> w392
      tunnel: w390 -> [w400 w434 w455 _ _ w526]
      tunnel: [w399 w418 w440 w464 w498 w519] -> w389
      tunnel: w388 -> [w398 w427 w448 w476 w508 w525]
      tunnel: w387 -> [_ _ _ w484 w515 _]
      tunnel: w386 -> [_ _ _ w477 w509 _]
      frame "Init", Default {
        n189 = case shown="False" w402 {
          tunnel: [AR-Auto-Purge."Init" ("Purge State") AR-Auto-Purge."Start Pump" ("Fill State")] -> w401
          tunnel: w400 -> [_ w413]
          tunnel: [errorcluster {"status"=FALSE, "code"=0, "source"=""} ("error out") w409] -> w399
          tunnel: w398 -> [_ w411]
          frame False {
          }
          frame True {
            w410 = FALSE
            w407 = T5."Disabled" ("Disabled")
            n190 = call "AR-Select-Single-DO.vi"("Action"=AR-DO-Action."Keep DO3") -> ("DO Data"=w412:bool[])  [unwired: 9 in, 1 out]
            n191 = call "AR-DO-write.vi"("error in (no error)"=w411, "Data"=w412, "DO task in"=w413) -> ("error out"=w409:errorcluster)  [unwired: 7 in, 1 out]
            n192 = local write "Purge Done"(FALSE ("Purge Done")) -> ()
            n193 = local write "Fill Done"(FALSE ("Purge Done")) -> ()
            n194 = property on="Pump (DO0)" class="Bool (strict)"(error in=w409, "DisabledEnum"=w407, "Value"=w410) -> ()  [unwired: 1 in, 2 out]
            n195 = property on="Vac sol (DO1)" class="Bool (strict)"("DisabledEnum"=w407, "Value"=w410) -> ()  [unwired: 2 in, 2 out]
            n196 = property on="Gas sol (DO2)" class="Bool (strict)"("DisabledEnum"=w407, "Value"=w410) -> ()  [unwired: 2 in, 2 out]
            n197 = property on="Auto fill" class="Bool (strict)"("DisabledEnum"=w407) -> ()  [unwired: 2 in, 2 out]
          }
        }
      }
      frame "Start Pump" {
        w415 = AR-DO-Action."Update" ("Action")
        w433 = TRUE ("DO")
        # "Auto Purge Turned Off"
        # "Pump ON"
        # "Vac SOL ON"
        n198 = local write "Vac SOL"(w433) -> ()
        n199 = call "AR-Select-Single-DO.vi"("Action"=w415, "DO"=w433, "index"=1) -> ("DO Data"=w435:bool[])  [unwired: 7 in, 1 out]
        n200 = call "AR-DO-write.vi"("error in (no error)"=w427, "Data"=w435, "DO task in"=w434) -> ("error out"=w428:errorcluster, "DO task out"=w431:refnum<k21>)  [unwired: 7 in]
        n201 = call "Time Delay"("error in (no error)"=w428) -> ("error out"=w417:errorcluster)  [unwired: 10 in]
        n202 = call "AR-Select-Single-DO.vi"("error in (no error)"=w417, "Action"=w415, "DO"=TRUE, "index"=0) -> ("error out"=w416:errorcluster, "DO Data"=w430:bool[])  [unwired: 6 in]
        n203 = call "AR-DO-write.vi"("error in (no error)"=w416, "Data"=w430, "DO task in"=w431) -> ("error out"=w421:errorcluster)  [unwired: 7 in, 1 out]
        n204 = property on="Pump (DO0)" class="Bool (strict)"(error in=w421, "Value"=TRUE ("Pump (DO0)")) -> (error out=w420:errorcluster)  [unwired: 1 in, 1 out]
        n205 = property on="Vac sol (DO1)" class="Bool (strict)"(error in=w420, "Value"=TRUE ("Vac sol (DO1)")) -> (error out=w418:errorcluster)  [unwired: 1 in, 1 out]
        n206 = Select(t=AR-Auto-Purge."10T Gage" ("Purge State"), s=w426, f=AR-Auto-Purge."End" ("Purge State")) -> (s? t:f=w423:T2)
      }
      frame "Stop Pump" {
        w437 = AR-DO-Action."Update" ("Action")
        w441 = FALSE ("Pump (DO0)")
        w454 = FALSE ("DO")
        # "Pump Off"
        # "Vac SOL Off"
        n207 = local write "Vac SOL"(w454) -> ()
        n208 = call "AR-Select-Single-DO.vi"("Action"=w437, "DO"=w454, "index"=1) -> ("DO Data"=w456:bool[])  [unwired: 7 in, 1 out]
        n209 = call "AR-DO-write.vi"("error in (no error)"=w448, "Data"=w456, "DO task in"=w455) -> ("error out"=w449:errorcluster, "DO task out"=w452:refnum<k21>)  [unwired: 7 in]
        n210 = call "Time Delay3"("error in (no error)"=w449) -> ("error out"=w439:errorcluster)  [unwired: 10 in]
        n211 = call "AR-Select-Single-DO.vi"("error in (no error)"=w439, "Action"=w437, "DO"=FALSE, "index"=0) -> ("error out"=w438:errorcluster, "DO Data"=w451:bool[])  [unwired: 6 in]
        n212 = call "AR-DO-write.vi"("error in (no error)"=w438, "Data"=w451, "DO task in"=w452) -> ("error out"=w443:errorcluster)  [unwired: 7 in, 1 out]
        n213 = property on="Pump (DO0)" class="Bool (strict)"(error in=w443, "Value"=w441) -> (error out=w442:errorcluster)  [unwired: 1 in, 1 out]
        n214 = property on="Vac sol (DO1)" class="Bool (strict)"(error in=w442, "Value"=w441) -> (error out=w440:errorcluster)  [unwired: 1 in, 1 out]
        n215 = Select(t=AR-Auto-Purge."1000T Gage" ("Purge State"), s=w447, f=AR-Auto-Purge."End") -> (s? t:f=w444:T2)
      }
      frame "10T Gage" {
        # "Auto Fill OFF"
        # "Vacuum reached"
        n216 = call "AR-DI-read.vi"("error in"=w476, "DI task in"=w477) -> ("error out"=w465:errorcluster, "Data"=w475:bool[])  [unwired: 7 in, 1 out]
        n217 = call "AR-AI-read.vi"("number of samples"=10, "error in"=w476, "AI task in"=w484) -> ("error out"=w466:errorcluster, "Data"=w483:dbl[])  [unwired: 6 in, 1 out]
        n218 = local read "simulate"() -> (w472:bool)
        n219 = Index Array(array=w475, index #1=0 ("index"), index #2=2 ("index")) -> (element #1=w471:bool)  [unwired: 1 out]
        n220 = Index Array(array=w483, index=0) -> (element=w481:dbl)
        n221 = Select(t="10T Sim 2", s=w472, f=w481) -> (s? t:f=w479:dbl)
        n222 = Select(t="<0.1T sim 2", s=w472, f=w471) -> (s? t:f=w469:bool)
        n223 = Less?(x=w479, y=0.1) -> (x < y?=w459:bool)
        n224 = Or(x=w469, y=w459) -> (x .or. y?=w458:bool)
        n225 = case shown="True" w458 {
          frame False {
          }
          frame True {
            n226 = One Button Dialog(message="Now it is safe to open the athmospheric valve to fill the chamber with air. ") -> ()  [unwired: 1 in, 1 out]
          }
        }
        n227 = Select(t=AR-Auto-Purge."Stop Pump" ("Purge State"), s=w458, f=AR-Auto-Purge."10T Gage") -> (s? t:f=w462:T2)
        n228 = Select(t=w462, s=w463, f=AR-Auto-Purge."End") -> (s? t:f=w460:T2)
        n229 = Merge Errors(w465, w466) -> (w464:errorcluster)
      }
      frame "1000T Gage" {
        # "Auto Purge OFF"
        n230 = call "AR-DI-read.vi"("error in"=w508, "DI task in"=w509) -> ("error out"=w499:errorcluster, "Data"=w507:bool[])  [unwired: 7 in, 1 out]
        n231 = call "AR-AI-read.vi"("number of samples"=10, "error in"=w508, "AI task in"=w515) -> ("error out"=w500:errorcluster, "Data"=w514:dbl[])  [unwired: 6 in, 1 out]
        n232 = local read "simulate"() -> (w504:bool)
        n233 = local read "Full Ar Limit Torr"() -> (w487:dbl)
        n234 = Index Array(array=w507, index #1=1 ("index"), index #2=2 ("index")) -> (element #1=w493:bool)  [unwired: 1 out]
        n235 = Index Array(array=w514, index=1) -> (element=w512:dbl)
        n236 = Not(x=">750 sim 2") -> (.not. x?=w490:bool)
        n237 = Not(x=w493) -> (.not. x?=w492:bool)
        n238 = Select(t="1000T Sim 2", s=w504, f=w512) -> (s? t:f=w510:dbl)
        n239 = Select(t=w490, s=w504, f=w492) -> (s? t:f=w503:bool)
        n240 = Greater Or Equal?(x=w510, y=w487) -> (x >= y?=w488:bool)
        n241 = Or(x=w503, y=w488) -> (x .or. y?=w489:bool)
        n242 = Select(t=AR-Auto-Purge."End" ("Purge State"), s=w489, f=AR-Auto-Purge."1000T Gage") -> (s? t:f=w496:T2)
        n243 = Select(t=w496, s=w497, f=AR-Auto-Purge."End") -> (s? t:f=w494:T2)
        n244 = Merge Errors(w499, w500) -> (w498:errorcluster)
      }
      frame "End" {
        w520 = T5."Enabled" ("Disabled")
        w522 = FALSE ("Vac SOL")
        w523 = FALSE
        n245 = call "AR-Select-Single-DO.vi"("Action"=AR-DO-Action."Keep DO3") -> ("DO Data"=w527:bool[])  [unwired: 9 in, 1 out]
        n246 = call "AR-DO-write.vi"("error in (no error)"=w525, "Data"=w527, "DO task in"=w526) -> ("error out"=w524:errorcluster)  [unwired: 7 in, 1 out]
        n247 = property on="Pump (DO0)" class="Bool (strict)"(error in=w524, "Value"=w523) -> (error out=w519:errorcluster)  [unwired: 1 in, 1 out]
        n248 = property on="Vac sol (DO1)" class="Bool (strict)"("Value"=w523) -> ()  [unwired: 2 in, 2 out]
        n249 = property on="Gas sol (DO2)" class="Bool (strict)"("Value"=w523) -> ()  [unwired: 2 in, 2 out]
        n250 = local write "Gas SOL"(w522) -> ()
        n251 = local write "Vac SOL"(w522) -> ()
        n252 = local write "O2 pwr"(w522) -> ()
        n253 = property on="Pump (DO0)" class="Bool (strict)"(error in=w519, "DisabledEnum"=w520) -> ()  [unwired: 1 in, 2 out]
        n254 = property on="Vac sol (DO1)" class="Bool (strict)"("DisabledEnum"=w520) -> ()  [unwired: 2 in, 2 out]
        n255 = property on="Gas sol (DO2)" class="Bool (strict)"("DisabledEnum"=w520) -> ()  [unwired: 2 in, 2 out]
        n256 = local write "Auto purge"(FALSE ("Auto purge")) -> ()
        n257 = property on="Auto fill" class="Bool (strict)"("DisabledEnum"=w520) -> ()  [unwired: 2 in, 2 out]
        "Purge Done" <- TRUE ("Fill Done")
      }
    }
    n258 = call "AR-GC-Stop-FGV.vi"("Action (RD)"=enum16{"Init", "WR", "RD"}."RD", "error in"=w389) -> ("error out"=w396:errorcluster, "Out"=w397:bool)  [unwired: 8 in]
    n259 = Compound Arithmetic op=OR(w397, w396) -> (w394:bool)
    "Purge State" <- w391
  }
  n260 = call "AR-GC-Stop-FGV.vi"("Action (RD)"=enum16{"Init", "WR", "RD"}."WR", "error in"=w12, "Action"=TRUE) -> ("error out"=w11:errorcluster)  [unwired: 7 in, 1 out]
  n261 = call "AR-DI-close.vi"("error in (no error)"=w11, "DI task in"=w23) -> ("error out"=w20:errorcluster)  [unwired: 9 in]
  n262 = call "AR-AI-close.vi"("error in (no error)"=w11, "AI task in"=w22) -> ("error out"=w19:errorcluster)  [unwired: 9 in]
  n263 = call "AR-DO-close.vi"("error in (no error)"=w11, "DO task in"=w24) -> ("error out"=w21:errorcluster)  [unwired: 9 in]
  n264 = Merge Errors(w21, w20, w19) -> (→"error out":errorcluster)
